vi "Launcher_PID.vi"() -> ()   [LabVIEW 2012]
uses:
  StateMachineEnum.ctl
  Robot Global Data.vi
panel:
  in  "PID gainsR":T1={"proportional gain (Kc)"=1.0, "integral time (Ti, min)"=0.01, "derivative time (Td, min)"=0.0} {"derivative time (Td, min)" format="%.3f"; "integral time (Ti, min)" format="%.3f"; "proportional gain (Kc)" format="%.3f"}
  in  "Output RangeR":cluster{"output high":dbl, "output low":dbl}={"output high"=100.0, "output low"=-100.0} {"output low" format="%.2f"; "output high" format="%.2f"}
  in  "PID gainsL":T1={"proportional gain (Kc)"=1.0, "integral time (Ti, min)"=0.01, "derivative time (Td, min)"=0.0} {"derivative time (Td, min)" format="%.3f"; "integral time (Ti, min)" format="%.3f"; "proportional gain (Kc)" format="%.3f"}
  in  "Output RangeL":cluster{"output high":dbl, "output low":dbl}={"output high"=100.0, "output low"=-100.0} {"output low" format="%.2f"; "output high" format="%.2f"}
  out "LoopInterval(ms)":u32
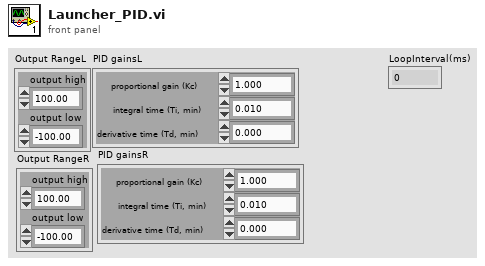
[diagram p1: front panel]
types:
  T1 = cluster{"proportional gain (Kc)":dbl, "integral time (Ti, min)":dbl, "derivative time (Td, min)":dbl}
  T2 = typedef "StateMachineEnum.ctl" = enum16{"Init", "Idle", "Start", "Do", "Stop"}
  T3 = typedef "WPI_EncoderDevRef.ctl" = cluster{"DevStatus":errorcluster, "EncoderIndex":T4, "CounterIndex":T5, "DistancePerCount":dbl, "Decoding Type":T6}
  T4 = typedef "FPGA_EncoderIdx.ctl" = enum8{"Enc 0", "Enc 1", "Enc 2", "Enc 3", "Invalid"}
  T5 = typedef "FPGA_CounterCtrSystemIndex.ctl" = enum8{"Ctr 0", "Ctr 1", "Ctr 2", "Ctr 3", "Ctr 4", "Ctr 5", "Ctr 6", "Ctr 7", "Invalid"}
  T6 = typedef "WPI_EncoderType.ctl" = enum16{"1x", "2x", "4x"}
  T7 = typedef "WPI_MotorControlDeviceRef.ctl" = cluster{"DeviceStatus":errorcluster, "Type":enum16{"PWM", "CAN"}, "PWM":cluster{"Digital Module":T8, "PWM Channel":T9, "DeadBand":T10}, "CAN":cluster{"Device Number":u8, "Control Mode":T11, "Semaphore":T12, "Max Vout":dbl}, "Invert":bool, "TransformRef":T13, "InvTransformRef":T13}
  T8 = typedef "FPGA_TypedefDigitalModule.ctl" = enum16{"Digital Module 1", "Digital Module 2"}
  T9 = typedef "FPGA_DIOPWMChannel.ctl" = enum8{"PWM 1", "PWM 2", "PWM 3", "PWM 4", "PWM 5", "PWM 6", "PWM 7", "PWM 8", "PWM 9", "PWM 10", "Invalid"}
  T10 = typedef "WPI_PWMDeadband.ctl" = cluster{"Name":string, "maxPositivePwm":i32, "minPositivePwm":i32, "centerPwm":i32, "maxNegativePwm":i32, "minNegativePwm":i32, "angularRange":u16}
  T11 = typedef "WPI_CANJaguar_ControlMode.ctl" = enum8{"Percent VBus", "Current", "Speed", "Position", "Voltage"}
  T12 = typedef "Semaphore RefNum" = refnum<k1>
  T13 = typedef "WPI_PWMTransform_ConPane.ctl" = refnum<vi>
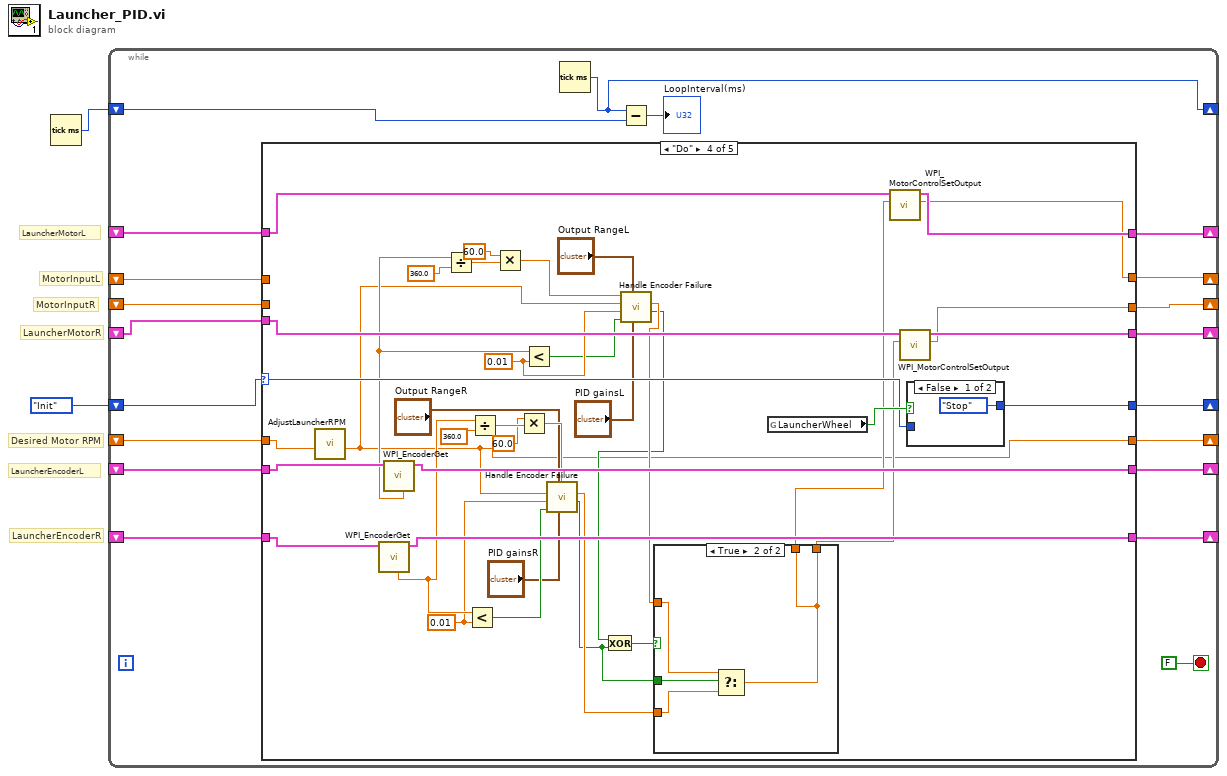
[diagram p0: block diagram]
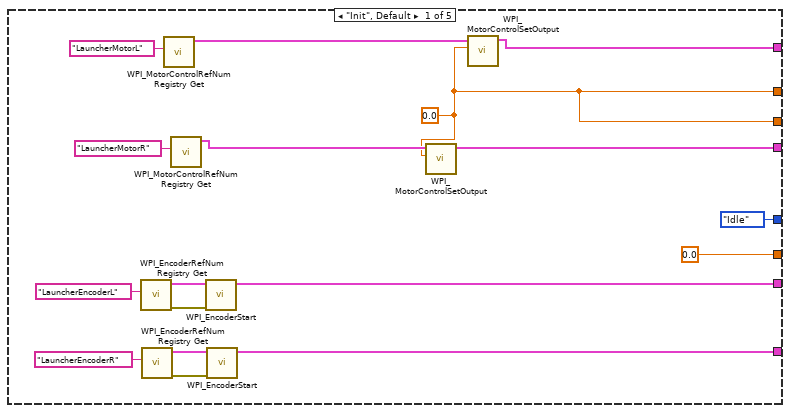
[diagram p2: hidden frame]
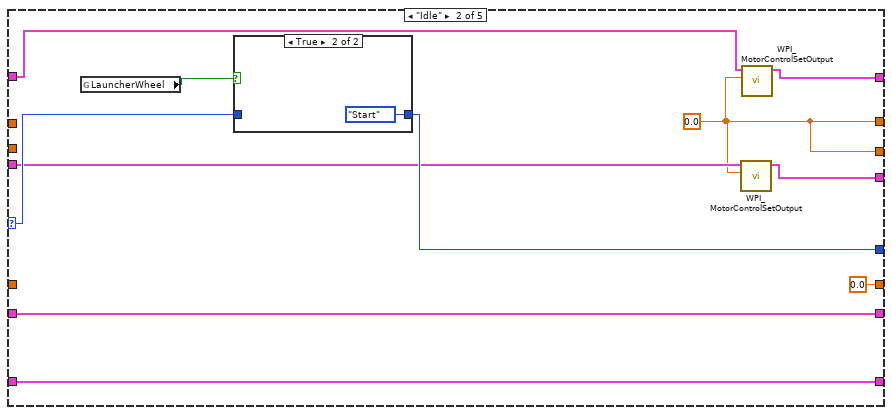
[diagram p3: hidden frame]
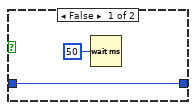
[diagram p4: hidden frame]
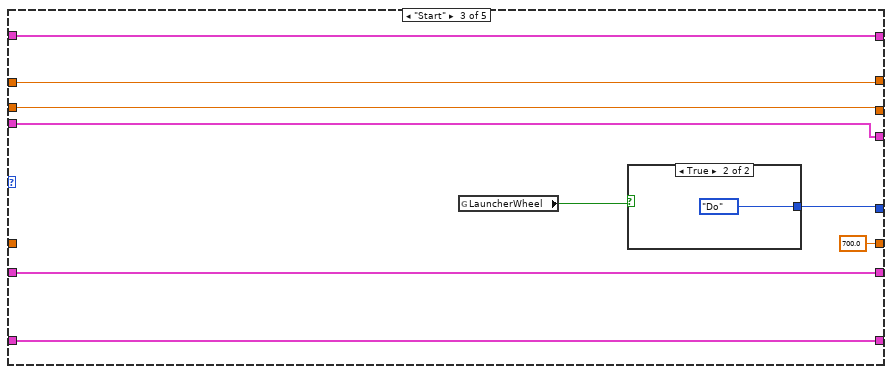
[diagram p5: hidden frame]
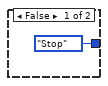
[diagram p6: hidden frame]
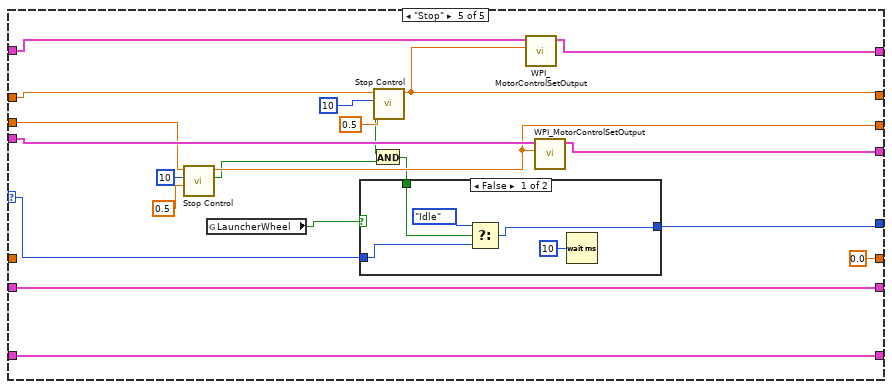
[diagram p9: hidden frame]
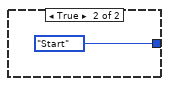
[diagram p10: hidden frame]
diagram:
  # "Desired Motor RPM"
  # "MotorInputR"
  # "LauncherEncoderR"
  # "LauncherEncoderL"
  # "LauncherMotorR"
  # "MotorInputL"
  # "LauncherMotorL"
  n1 = Tick Count (ms)() -> (millisecond timer value=w1:u32)
  n2 = while {
    shift-right: [w19] -> _
    shift-left: w1 -> [w20]
    shift-right: [w17] -> _
    shift-left: _ -> [w11]
    shift-right: [w16] -> _
    shift-left: _ -> [w7]
    shift-right: [w15] -> _
    shift-left: _ -> [w10]
    shift-right: [w14] -> _
    shift-left: _ -> [w9]
    shift-right: [w13] -> _
    shift-left: _ -> [w8]
    shift-right: [w12] -> _
    shift-left: StateMachineEnum."Init" ("State") -> [w21]
    shift-right: [w6] -> _
    shift-left: _ -> [w5]
    shift-right: [w4] -> _
    shift-left: _ -> [w3]
    stop <- FALSE stop-if-true
    n3 = case shown="\"Do\"" w21 {
      selector: w21 -> [_ w49 _ w89 w121]
      tunnel: [w37 w46 w60 w102 w129] -> w17
      tunnel: [w24 w40 w62 w67 w127] -> w16
      tunnel: [w34 w47 w61 w104 w130] -> w15
      tunnel: [w27 w43 w59 w98 w132] -> w14
      tunnel: [w26 w42 w58 w100 w133] -> w13
      tunnel: [StateMachineEnum."Idle" ("State") w48 w56 w88 w122] -> w12
      tunnel: w11 -> [_ w45 w60 w103 w128]
      tunnel: w10 -> [_ w44 w61 w91 w131]
      tunnel: w9 -> [_ w43 w59 w99 w132]
      tunnel: w8 -> [_ w42 w58 w101 w133]
      tunnel: w7 -> [_ _ w62 _ w126]
      tunnel: [w24 w40 w55 w66 w119] -> w6
      tunnel: w5 -> [_ _ w55 _ w120]
      tunnel: [0.0 0.0 700.0 w65 0.0 ("New RPM")] -> w4
      tunnel: w3 -> [_ _ _ w86 _]
      frame "Init", Default {
        w24 = 0.0 ("Output")
        n4 = call <vilib>:"WPI_EncoderRefNum Registry Get.vi"("refnum name"="LauncherEncoderL") -> ("error out"=w32:errorcluster, "EncoderDevRef"=w33:T3)  [unwired: 9 in]
        n5 = call <vilib>:"WPI_EncoderRefNum Registry Get.vi"("refnum name"="LauncherEncoderR") -> ("error out"=w29:errorcluster, "EncoderDevRef"=w30:T3)  [unwired: 9 in]
        n6 = call <vilib>:"WPI_MotorControlRefNum Registry Get.vi"("refnum name"="LauncherMotorL") -> ("MotorControlDevRef"=w38:T7)  [unwired: 9 in, 1 out]
        n7 = call <vilib>:"WPI_MotorControlRefNum Registry Get.vi"("refnum name"="LauncherMotorR") -> ("MotorControlDevRef"=w35:T7)  [unwired: 9 in, 1 out]
        n8 = call <vilib>:"WPI_EncoderStart.vi"("error in (no error)"=w32, "EncoderDevRef"=w33) -> ("EncoderDevRef"=w27:T3)  [unwired: 8 in, 1 out]
        n9 = call <vilib>:"WPI_EncoderStart.vi"("error in (no error)"=w29, "EncoderDevRef"=w30) -> ("EncoderDevRef"=w26:T3)  [unwired: 8 in, 1 out]
        n10 = call <vilib>:"WPI_MotorControlSetOutput.vi"("Output"=w24, "MotorControlDevRef"=w35) -> ("MotorControlDevRef"=w34:T7)  [unwired: 7 in, 2 out]
        n11 = call <vilib>:"WPI_MotorControlSetOutput.vi"("Output"=w24, "MotorControlDevRef"=w38) -> ("MotorControlDevRef"=w37:T7)  [unwired: 7 in, 2 out]
      }
      frame "Idle" {
        w40 = 0.0 ("Output")
        n12 = global read "Robot Global Data.vi" "LauncherWheel"() -> (w50:bool)
        n13 = case shown="True" w50 {
          tunnel: w49 -> [w52 _]
          tunnel: [w52 StateMachineEnum."Start" ("State")] -> w48
          frame False {
            n14 = Wait (ms)(milliseconds to wait=u32 50) -> ()  [unwired: 1 out]
          }
          frame True {
          }
        }
        n15 = call <vilib>:"WPI_MotorControlSetOutput.vi"("Output"=w40, "MotorControlDevRef"=w44) -> ("MotorControlDevRef"=w47:T7)  [unwired: 7 in, 2 out]
        n16 = call <vilib>:"WPI_MotorControlSetOutput.vi"("Output"=w40, "MotorControlDevRef"=w45) -> ("MotorControlDevRef"=w46:T7)  [unwired: 7 in, 2 out]
      }
      frame "Start" {
        n17 = global read "Robot Global Data.vi" "LauncherWheel"() -> (w57:bool)
        n18 = case shown="True" w57 {
          tunnel: [StateMachineEnum."Stop" ("State") StateMachineEnum."Do" ("State")] -> w56
          frame False {
          }
          frame True {
          }
        }
      }
      frame "Do" {
        w80 = 0.01 ("y")
        w79 = 0.01 ("y")
        n19 = call "AdjustLauncherRPM.vi"("Current RPM"=w86) -> ("New RPM"=w65:dbl)  [unwired: 10 in]
        n20 = call <vilib>:"WPI_EncoderGet.vi"("EncoderDevRef"=w101) -> ("EncoderDevRef"=w100:T3, "Rate"=w82:dbl)  [unwired: 5 in, 4 out]
        n21 = call <vilib>:"WPI_EncoderGet.vi"("EncoderDevRef"=w99) -> ("EncoderDevRef"=w98:T3, "Rate"=w81:dbl)  [unwired: 5 in, 4 out]
        n22 = Divide(x=w81, y=360.0) -> (x/y=w95:dbl)
        n23 = Less?(x=w82, y=w80) -> (x < y?=w78:bool)
        n24 = Divide(x=w82, y=360.0) -> (x/y=w94:dbl)
        n25 = Multiply(x=60.0, y=w95) -> (x*y=w85:dbl)
        n26 = Multiply(x=60.0, y=w94) -> (x*y=w87:dbl)
        n27 = Less?(x=w81, y=w79) -> (x < y?=w77:bool)
        n28 = call "Handle Encoder Failure.vi"("PID gains"="PID gainsR", "Output Range"="Output RangeR", "Encoder Failure"=w78, "Loop Time"=w80, "Desired RPM"=w65, "Current RPM"=w87) -> ("Encoder Failure Out"=w74:bool, "Motor Output"=w84:dbl)  [unwired: 4 in]
        n29 = call "Handle Encoder Failure.vi"("PID gains"="PID gainsL", "Output Range"="Output RangeL", "Encoder Failure"=w77, "Loop Time"=w79, "Desired RPM"=w65, "Current RPM"=w85) -> ("Encoder Failure Out"=w76:bool, "Motor Output"=w83:dbl)  [unwired: 4 in]
        n30 = Exclusive Or(1:w74, 2:w76) -> (0:w75:bool)
        n31 = case shown="True" w75 {
          tunnel: w84 -> [w105 w109]
          tunnel: w83 -> [w106 w108]
          tunnel: w74 -> [_ w110]
          tunnel: [w105 w107] -> w73
          tunnel: [w106 w107] -> w72
          frame False {
          }
          frame True {
            n32 = Select(t=w108, s=w110, f=w109) -> (s? t:f=w107:dbl)
          }
        }
        n33 = global read "Robot Global Data.vi" "LauncherWheel"() -> (w90:bool)
        n34 = call <vilib>:"WPI_MotorControlSetOutput.vi"("Output"=w72, "MotorControlDevRef"=w103) -> ("Motor Output"=w67:dbl, "MotorControlDevRef"=w102:T7)  [unwired: 7 in, 1 out]
        n35 = call <vilib>:"WPI_MotorControlSetOutput.vi"("Output"=w73, "MotorControlDevRef"=w91) -> ("Motor Output"=w66:dbl, "MotorControlDevRef"=w104:T7)  [unwired: 7 in, 1 out]
        n36 = case shown="False" w90 {
          tunnel: w89 -> [_ w112]
          tunnel: [StateMachineEnum."Stop" ("State") w112] -> w88
          frame False {
          }
          frame True {
          }
        }
      }
      frame "Stop" {
        n37 = call "Stop Control.vi"("Rate (unit/s)"=0.5, "Loop Time (ms)"=u32 10, "Recieved Motor Input"=w120) -> ("Done Stopping"=w116:bool, "New Motor Input"=w119:dbl)  [unwired: 7 in]
        n38 = global read "Robot Global Data.vi" "LauncherWheel"() -> (w123:bool)
        n39 = call "Stop Control.vi"("Rate (unit/s)"=0.5, "Loop Time (ms)"=u32 10, "Recieved Motor Input"=w126) -> ("Done Stopping"=w115:bool, "New Motor Input"=w127:dbl)  [unwired: 7 in]
        n40 = And(x=w115, y=w116) -> (x .and. y?=w114:bool)
        n41 = case shown="False" w123 {
          tunnel: [w137 StateMachineEnum."Start" ("State")] -> w122
          tunnel: w121 -> [w138 _]
          tunnel: w114 -> [w134 _]
          frame False {
            n42 = Select(t=StateMachineEnum."Idle", s=w134, f=w138) -> (s? t:f=w137:T2)
            n43 = Wait (ms)(milliseconds to wait=u32 10) -> ()  [unwired: 1 out]
          }
          frame True {
          }
        }
        n44 = call <vilib>:"WPI_MotorControlSetOutput.vi"("Output"=w127, "MotorControlDevRef"=w128) -> ("MotorControlDevRef"=w129:T7)  [unwired: 7 in, 2 out]
        n45 = call <vilib>:"WPI_MotorControlSetOutput.vi"("Output"=w119, "MotorControlDevRef"=w131) -> ("MotorControlDevRef"=w130:T7)  [unwired: 7 in, 2 out]
      }
    }
    n46 = Tick Count (ms)() -> (millisecond timer value=w19:u32)
    n47 = Subtract(x=w19, y=w20) -> (x-y=→"LoopInterval(ms)":u32)
  }
